vi "Digital Read Benchmark.vi"() -> ()   [LabVIEW 2013]
uses:
  <vilib>/LabVIEW Hacker/LINX/Private/Type Defs/Interface.ctl
  <vilib>/LabVIEW Hacker/LINX/Private/Device/Device.lvlib
  <vilib>/LabVIEW Hacker/LINX/LVH-LINX.lvlib
  <vilib>/ptbypt/NI_PtbyPt.lvlib
panel:
  out "Device Name":string
  out "Values":bool[](array[boolean])
  in  "DIO Channels":u8[](array[numeric])
  out "Loop Time (ms)":i32
  out "Loop Rate":dbl(graph)
  in  "Stop Button":bool
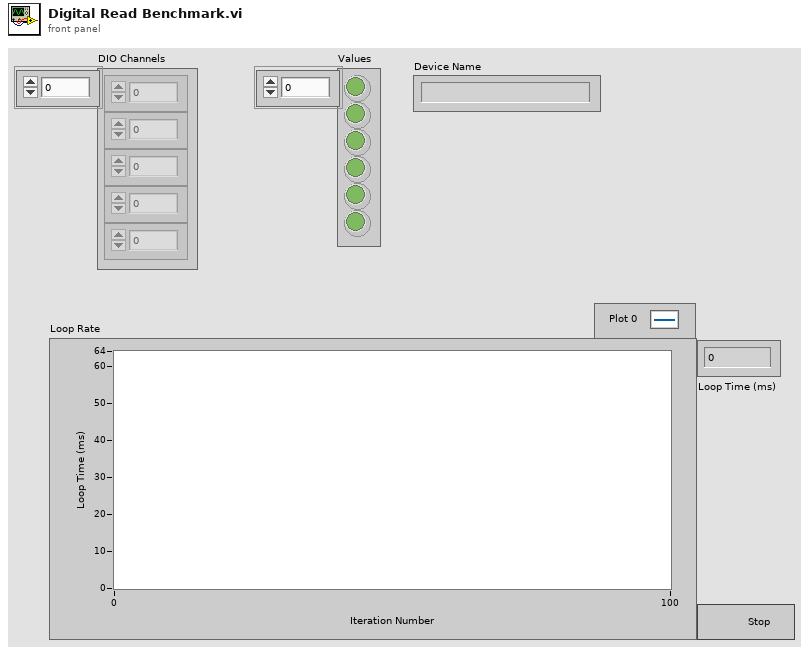
[diagram p1: front panel]
types:
  T1 = typedef "LVH-LINX.lvlib/Interface.ctl" = enum16{"Serial", "TCP"}
  T2 = typedef "LVH-LINX.lvlib/Device.lvlib/LINX Device Config.ctl" = cluster{"Interface":T1, "COM Port":refnum<visa-resource-name>, "TCP Configuration":T3, "Device Family":T4, "Device ID":u8, "Device Name":string, "TCP Ref":refnum<k5>}
  T3 = typedef "LVH-LINX.lvlib/Device.lvlib/TCP Config.ctl" = cluster{"IP Address":string, "Port":u16}
  T4 = typedef "LVH-LINX.lvlib/Device Family.ctl" = enum8{"National Instruments", "Digilent", "Arduino"}
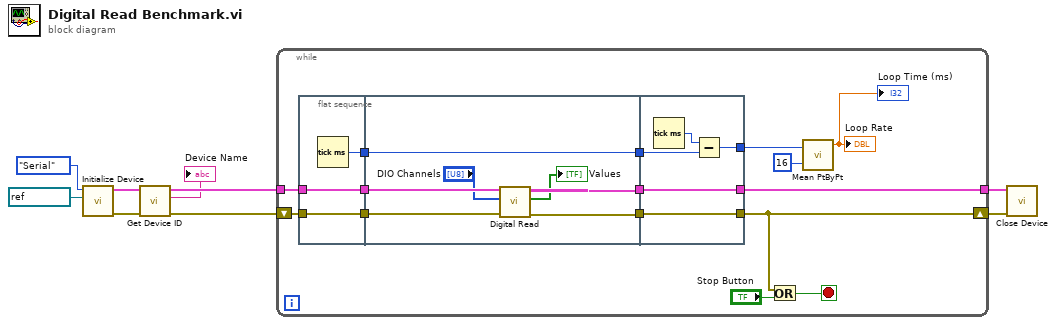
[diagram p0: block diagram]
diagram:
  n1 = call <vilib>:"Initialize Device.vi"("COM Port"=refnum<visa-resource-name> "COM5", "Interface"=Interface."Serial") -> ("Error Out"=w4:errorcluster, "LINX Device Config"=w5:T2)  [unwired: 7 in, 1 out]
  n2 = call <vilib>:"Get Device ID.vi"("Error In"=w4, "LINX Device Config"=w5) -> ("Error Out"=w3:errorcluster, "Device Name"=→"Device Name":string, "LINX Device Config"=w2:T2)  [unwired: 7 in]
  n3 = while {
    tunnel: w2 -> [w23]
    tunnel: [w22] -> w6
    shift-right: [w20] -> w7
    shift-left: w3 -> [w24]
    stop <- w21 stop-if-true
    n4 = flat-sequence {
      tunnel: w23 -> [w26]
      tunnel: w24 -> [w27]
      tunnel: [w27] -> w18
      tunnel: [w26] -> w17
      tunnel: [w25] -> w14
      tunnel: w18 -> [w30]
      tunnel: w17 -> [w33]
      tunnel: [w32] -> w16
      tunnel: [w31] -> w15
      tunnel: w14 -> [w34]
      tunnel: [w34] -> w13
      tunnel: [w38] -> w20
      tunnel: [w39] -> w22
      tunnel: w16 -> [w39]
      tunnel: w15 -> [w38]
      tunnel: w13 -> [w36]
      tunnel: [w35] -> w12
      frame #0 {
        n5 = Tick Count (ms)() -> (millisecond timer value=w25:u32)
      }
      frame #1 {
        n6 = call <vilib>:"Digital Read.vi"("Error In"=w30, "DIO Channels"="DIO Channels", "LINX Device Config"=w33) -> ("Error Out"=w31:errorcluster, "Values"=→"Values":bool[], "LINX Device Config"=w32:T2)  [unwired: 6 in]
      }
      frame #2 {
        n7 = Tick Count (ms)() -> (millisecond timer value=w37:u32)
        n8 = Subtract(x=w37, y=w36) -> (x-y=w35:u32)
      }
    }
    n9 = Or(x=w20, y="Stop Button") -> (x .or. y?=w21:bool)
    n10 = call <vilib>:"Mean PtByPt.vi"("x"=w12, "sample length"=16) -> ("mean"=→"Loop Rate" →"Loop Time (ms)":dbl)  [unwired: 2 in, 1 out]
  }
  n11 = call <vilib>:"Close Device.vi"("Error In"=w7, "LINX Device Config"=w6) -> ()  [unwired: 8 in, 2 out]
